vi "DynamicMotionMagicVoltage Setter.vi"(0 "LimitReverseMotion":bool, 1 "Acceleration":dbl, 2 "EnableFOC":bool=TRUE, 3 "Update Frequency (Hz)":dbl=100.0, 5 "StopSendingOtherRequests":bool=TRUE, 7 "Position":dbl, 9 "Velocity":dbl, 12 "Jerk":dbl, 13 "FeedForward":dbl) -> (4 "DeviceReference Out":T1)   [LabVIEW 2023]
doc: "Requests Motion Magic® to target a final position using a motion profile. This dynamic request allows runtime changes to Cruise Velocity, Acceleration, and Jerk. Users can optionally provide a voltage feedforward. This control requires use of a CANivore.\nMotion Magic® produces a motion profile in real-time while attempting to honor the specified Cruise Velocity, Acceleration, and Jerk value. This control mode does not use the Expo_kV or Expo_kA configs. Target position can be changed on-the-fly and Motion Magic® will do its best to adjust the profile. This control mode is voltage-based, so relevant closed-loop gains will use Volts for the numerator."
uses:
  Users/Cory/Documents/PhoenixPro-LabVIEW-Generation/controls/DeviceReference.ctl
panel:
  in  "LimitForwardMotion":bool
  in  "OverrideBrakeDurNeutral":bool
  in  "Slot":i32
  in  "DeviceReference":T1
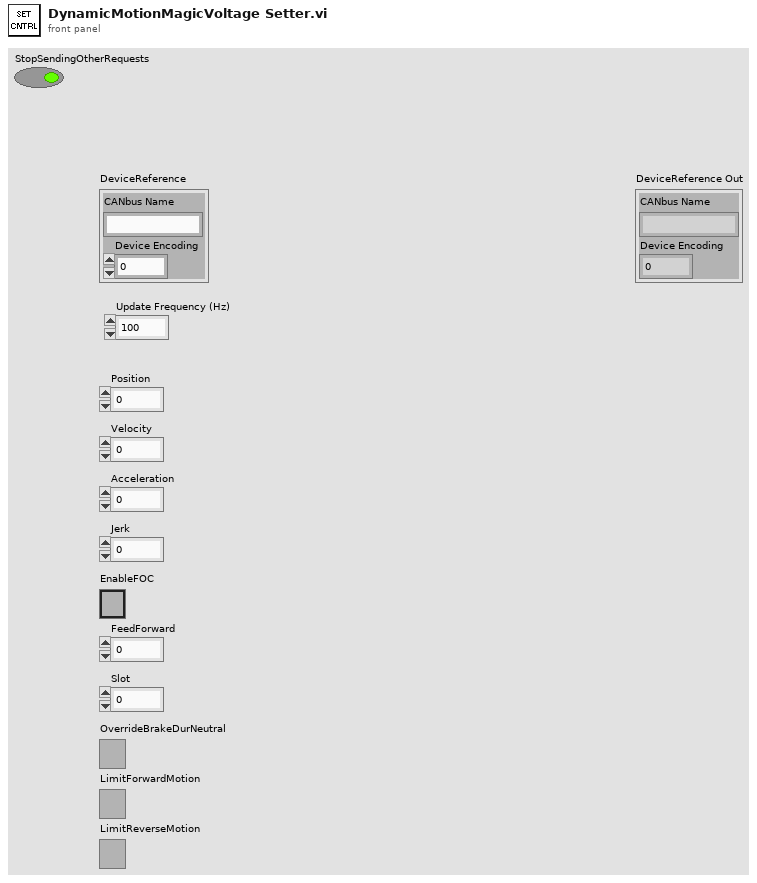
[diagram p1: front panel]
types:
  T1 = typedef "DeviceReference.ctl" = cluster{"CANbus Name":string, "Device Encoding":u32}
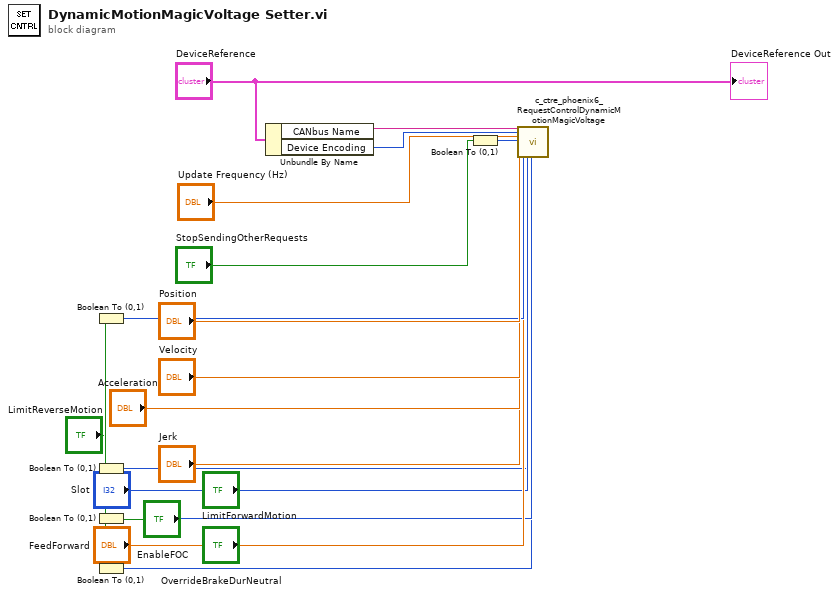
[diagram p0: block diagram]
diagram:
  n1 = Boolean To (0,1)(Boolean="EnableFOC") -> (0, 1=w9:i16)
  n2 = Boolean To (0,1)(Boolean="OverrideBrakeDurNeutral") -> (0, 1=w5:i16)
  n3 = Boolean To (0,1)(Boolean="LimitForwardMotion") -> (0, 1=w3:i16)
  n4 = Boolean To (0,1)(Boolean="LimitReverseMotion") -> (0, 1=w1:i16)
  n5 = Unbundle By Name("DeviceReference") -> ("CANbus Name"=w19:string, "Device Encoding"=w18:u32)
  n6 = Boolean To (0,1)(Boolean="StopSendingOtherRequests") -> (0, 1=w15:i16)
  n7 = call <vilib>:"c_ctre_phoenix6_RequestControlDynamicMotionMagicVoltage.vi"("String"=w19, "Numeric 2"=w18, "Numeric 3"="Update Frequency (Hz)", "Numeric 4"=w15, "Numeric 5"="Position", "Numeric 6"="Velocity", "Numeric 7"="Acceleration", "Numeric 8"="Jerk", "Numeric 9"=w9, "Numeric 10"="FeedForward", "Numeric 11"="Slot", "Numeric 12"=w5, "Numeric 13"=w3, "Numeric 14"=w1) -> ()  [unwired: 13 in, 1 out]
  "DeviceReference Out" <- "DeviceReference"
